vi "Home Stage.vi"(8 "error in (no error)":errorcluster, 11 "Stage Actor.lvlib:Stage.lvclass":refnum<class "Stage.lvclass">) -> (0 "error out":errorcluster, 3 "Stage Actor.lvlib:Stage.lvclass":refnum<class "Stage.lvclass">)   [LabVIEW 2018, in "Stage Actor.lvlib" / "Stage.lvclass"]
uses:
  Stage.lvclass
  Stage.lvclass/Stage.ctl
  <instrlib>/Zaber A Series/Zaber A Series.lvlib
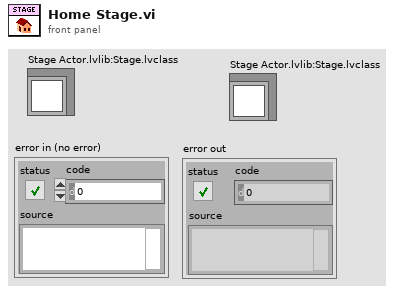
[diagram p1: front panel]
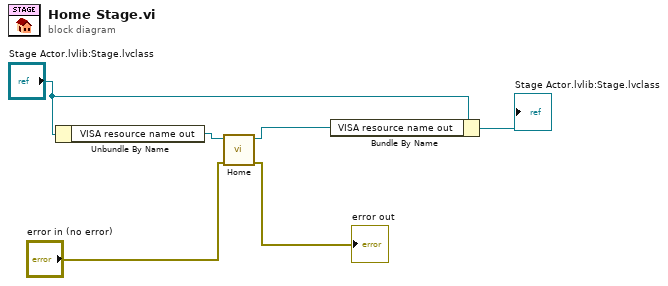
[diagram p0: block diagram]
diagram:
  n1 = Unbundle By Name("Stage Actor.lvlib:Stage.lvclass") -> ("VISA resource name out"=w6:refnum<visa-resource-name>)
  n2 = call <instrlib>:"Home.vi"("error in (no error)"="error in (no error)", "VISA resource name"=w6) -> ("error out"=→"error out":errorcluster, "VISA resource name out"=w1:refnum<visa-resource-name>)  [unwired: 8 in]
  n3 = Bundle By Name(cluster="Stage Actor.lvlib:Stage.lvclass", "VISA resource name out"=w1) -> (→"Stage Actor.lvlib:Stage.lvclass":refnum<class "Stage.lvclass">)
